vi "Element of Set.vi"(0 "DBSet in":refnum<class "DBSet.lvclass">, 5 "Element":string, 11 "error in (no error)":errorcluster {"code" format="Error %.0f"}) -> (4 "DBSet out":refnum<class "DBSet.lvclass">, 6 "Found?":bool, 15 "error out":errorcluster {"code" format="Error %.0f"})   [LabVIEW 2024, in "DBSet.lvclass"]
uses:
  DBSet.lvclass
  DBSet.lvclass/DBSet.ctl
  <vilib>/drjdpowell/SQLite Library/SQLite.lvlib
  <vilib>/drjdpowell/SQLite Library/SQL Connection/Execute SQL (Single Integer).vi
  <vilib>/drjdpowell/SQLite Library/SQL Connection/Connection.lvclass
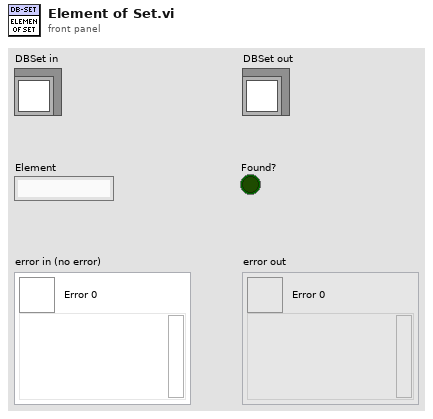
[diagram p1: front panel]
types:
  T1 = typedef "Semaphore RefNum" = refnum<k1>
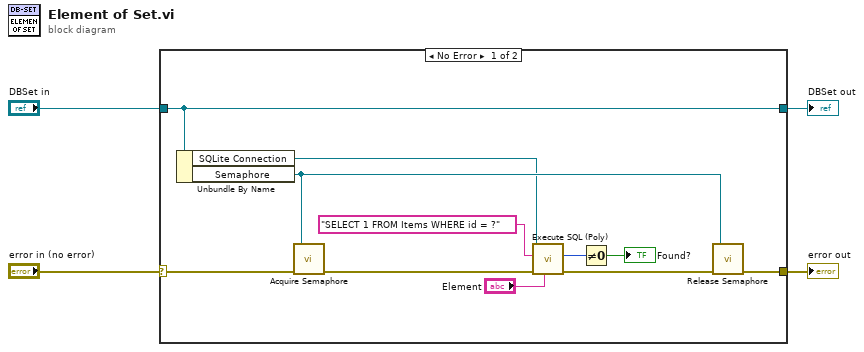
[diagram p0: block diagram]
diagram:
  n1 = case shown="No Error" "error in (no error)" {
    selector: "error in (no error)" -> [w14 w17]
    tunnel: [w13 w17] -> w3
    tunnel: [w15 w16] -> w1
    tunnel: "DBSet in" -> [w15 w16]
    frame No Error {
      n2 = Unbundle By Name(w15) -> ("SQLite Connection"=w5:refnum<class "Connection.lvclass">, "Semaphore"=w12:T1)
      n3 = call <vilib>:"Acquire Semaphore.vi"("error in (no error)"=w14, "semaphore"=w12) -> ("error out"=w7:errorcluster)  [unwired: 3 in, 2 out]
      n4 = call-poly <vilib>:"Execute SQL (Poly).vi"("Parameter(s)"="Element", "error in (no error)"=w7, "SQL"="SELECT 1 FROM Items WHERE id = ?", "SQLite Connection in"=w5) -> ("error out"=w6:errorcluster, "Result"=w9:i64)  [unwired: 5 in, 1 out]
      n5 = Not Equal To 0?(x=w9) -> (x != 0?=→"Found?":bool)
      n6 = call <vilib>:"Release Semaphore.vi"("error in (no error)"=w6, "semaphore"=w12) -> ("error out"=w13:errorcluster)  [unwired: 4 in, 1 out]
    }
    frame Error {
    }
  }
  "error out" <- w3
  "DBSet out" <- w1
